vi "Read Azimuth.vi"(8 "error in (no error)":errorcluster, 11 "MccAzElMove in":refnum<class "MccAzElMove.lvclass">) -> (0 "error out":errorcluster, 2 "azimuth":dbl[unit] min=0.0 max=6.283185132646661, 3 "MccAzElMove out":refnum<class "MccAzElMove.lvclass">)   [LabVIEW 2014, in "TCSDataDefinitions.lvlib" / "TCSMountControlCommand.lvlib" / "CommandsForAzElAxes.lvlib" / "MccAzElMove.lvclass"]
uses:
  MccAzElMove.lvclass
  MccAzElMove.lvclass/MccAzElMove.ctl
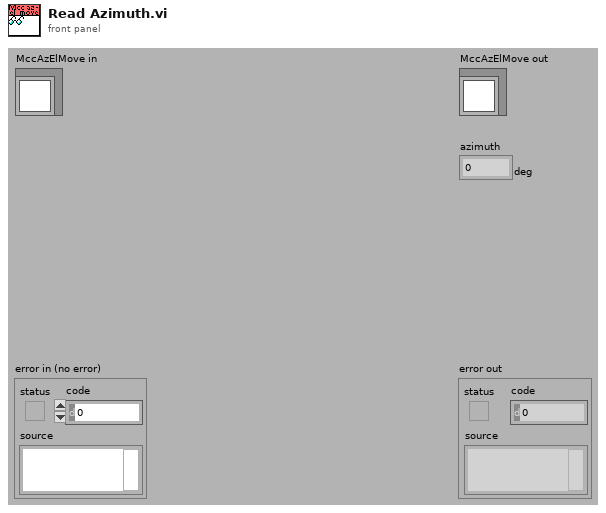
[diagram p1: front panel]
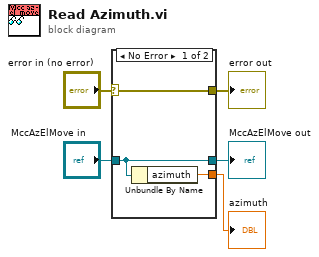
[diagram p0: block diagram]
diagram:
  n1 = case shown="No Error" "error in (no error)" {
    selector: "error in (no error)" -> [w8 w9]
    tunnel: [w8 w9] -> w4
    tunnel: [w7 w10] -> w2
    tunnel: "MccAzElMove in" -> [w7 w10]
    tunnel: [w6 _] -> w1
    frame No Error {
      n2 = Unbundle By Name(w7) -> ("azimuth"=w6:dbl[unit])
    }
    frame Error {
    }
  }
  "error out" <- w4
  "MccAzElMove out" <- w2
  "azimuth" <- w1
